vi "Get_reference_samplingdata.vi"(0 "SPU":refnum<k24>, 1 "STSProcess.ILSTS":refnum<k24>, 2 "Refdata_struct":refnum<k24>[](array[refnum]), 5 "Ref_monitordata_struct":refnum<k24>[](array[refnum]), 7 "MPM":refnum<k24>[](array[refnum]), 11 "错误输入（无错误）":errorcluster) -> (6 "ILSTS out":refnum<k24>, 15 "error out":errorcluster)   [LabVIEW 2017]
doc: "Get logging reference data & add in"
uses:
  D:/test/ILSTS/LV_IL_Sample/DLL/STSProcess.dll
  DLL/STSProcess.dll
  D:/test/ILSTS/LV_IL_Sample/DLL/InstrumentDLL.dll
  DLL/InstrumentDLL.dll
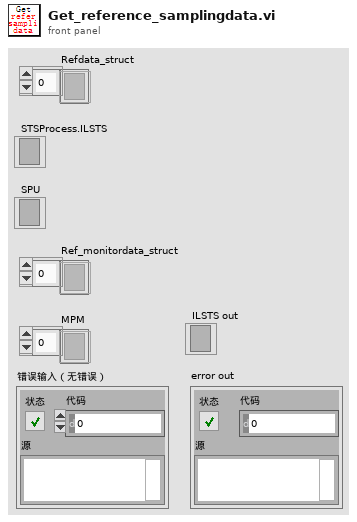
[diagram p1: front panel]
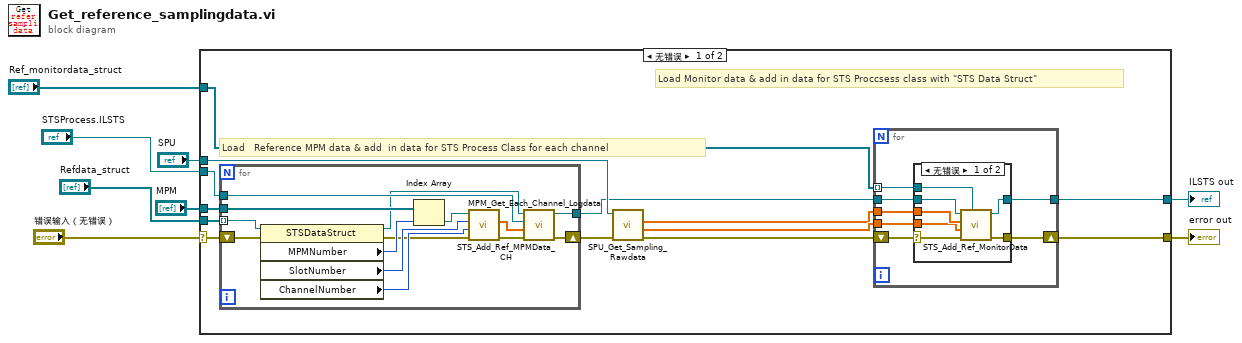
[diagram p0: block diagram]
diagram:
  n1 = case shown="无错误" "错误输入（无错误）" {
    selector: "错误输入（无错误）" -> [w12 w53]
    tunnel: "STSProcess.ILSTS" -> [w11 w52]
    tunnel: "Ref_monitordata_struct" -> [w18 _]
    tunnel: "SPU" -> [w17 _]
    tunnel: "MPM" -> [w15 _]
    tunnel: "Refdata_struct" -> [w14 _]
    tunnel: [w13 w53] -> w3
    tunnel: [w9 w52] -> w1
    frame No Error {
      # "Load Monitor data & add in data for STS Proccsess class with \"STS Data Struct\""
      # "Load　Reference MPM data & add  in data for STS Process Class for each channel"
      n2 = for {
        tunnel: w14 -> [w46] mode=indexing
        tunnel: w15 -> [w49]
        tunnel: w11 -> [w47]
        shift-right: [w45] -> w16
        shift-left: w12 -> [w43]
        tunnel: [w38] -> w10
        n3 = property on="属性节点" class="STSDataStruct"(reference=w46, error in=w43) -> (reference out=w39:refnum<k24>, error out=w44:errorcluster, "MPMNumber"=w48:i32, "SlotNumber"=w51:i32, "ChannelNumber"=w50:i32)
        n4 = Index Array(array=w49, index=w48) -> (element=w42:refnum<k24>)
        n5 = call "MPM_Get_Each_Channel_Logdata.vi"("error in (no error)"=w44, "channelNumber"=w50, "moduleNumber"=w51, ".NET Reference in"=w42) -> ("error out"=w40:errorcluster, "data out"=w41:sgl[])  [unwired: 5 in, 1 out]
        n6 = call "STS_Add_Ref_MPMData_CH.vi"("错误输入（无错误）"=w40, "data"=w41, "STSProcess.ILSTS"=w47, "Setting"=w39) -> ("错误输出"=w45:errorcluster, "ILSTS"=w38:refnum<k24>)  [unwired: 6 in]
      }
      n7 = call "SPU_Get_Sampling_Rawdata.vi"("错误输入（无错误）"=w16, "SPU"=w17) -> ("error out"=w19:errorcluster, "monitor"=w21:sgl[], "trigger"=w20:sgl[])  [unwired: 5 in, 1 out]
      n8 = for {
        tunnel: w18 -> [w27] mode=indexing
        tunnel: w10 -> [w28]
        tunnel: w20 -> [w26]
        tunnel: w21 -> [w25]
        shift-right: [w23] -> w13
        shift-left: w19 -> [w24]
        tunnel: [w22] -> w9
        n9 = case shown="无错误" w24 {
          selector: w24 -> [w31 w37]
          tunnel: w28 -> [w35 w36]
          tunnel: w27 -> [w34 _]
          tunnel: w26 -> [w33 _]
          tunnel: w25 -> [w32 _]
          tunnel: [w30 w37] -> w23
          tunnel: [w29 w36] -> w22
          frame No Error {
            n10 = call "STS_Add_Ref_MonitorData.vi"("setting"=w34, "错误输入（无错误）"=w31, "monitorData"=w32, "triggerIndex"=w33, "STSProcess.ILSTS"=w35) -> ("错误输出"=w30:errorcluster, "ILSTS out"=w29:refnum<k24>)  [unwired: 5 in]
          }
          frame Error {
          }
        }
      }
    }
    frame Error {
    }
  }
  "error out" <- w3
  "ILSTS out" <- w1
